vi "compile_table.vi"(6 "income_array":dbl[][](array[numeric]), 7 "row_number":i32, 8 "error_in":errorcluster, 9 "value":dbl, 10 "boc-data":sgl[](array[numeric]), 11 "measured":dbl[](array[numeric])) -> (0 "error_out":errorcluster, 2 "table":string[][](array[string]), 3 "output_data":dbl[][](array[numeric]))   [LabVIEW 2017]
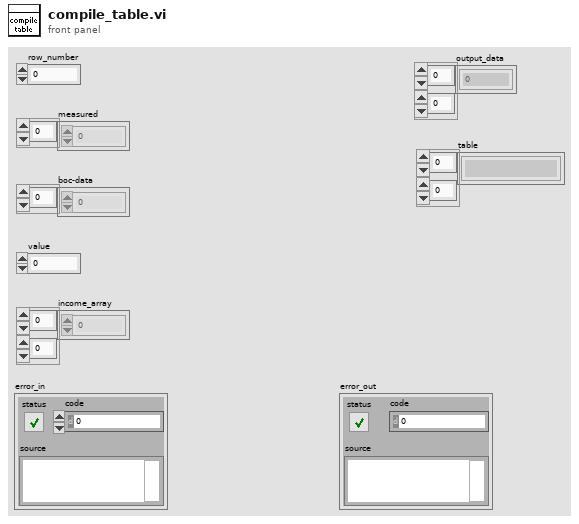
[diagram p1: front panel]
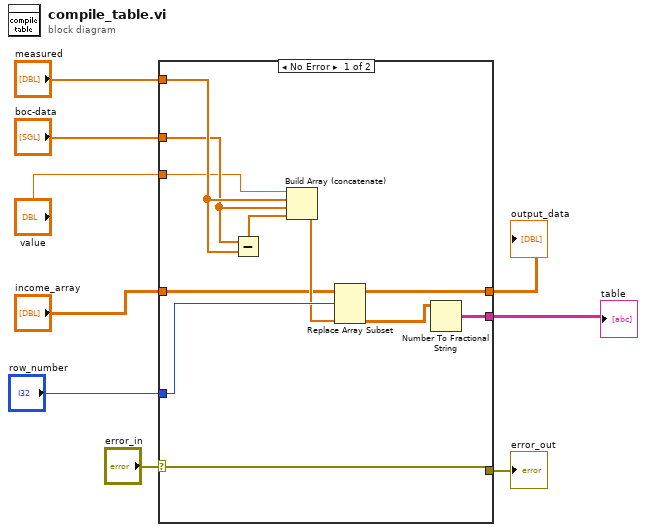
[diagram p0: block diagram]
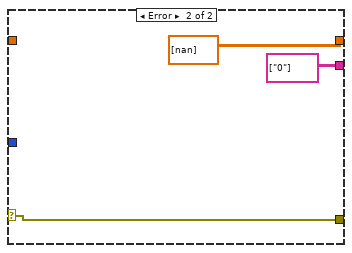
[diagram p2: hidden frame]
diagram:
  n1 = case shown="No Error" "error_in" {
    selector: "error_in" -> [w12 w22]
    tunnel: "measured" -> [w19 _]
    tunnel: "boc-data" -> [w18 _]
    tunnel: "row_number" -> [w16 _]
    tunnel: [w10 dbl[][] [[nan]] ("income_array")] -> w6
    tunnel: [w11 string[][] [["0"]]] -> w5
    tunnel: "income_array" -> [w14 _]
    tunnel: "value" -> [w13 _]
    tunnel: [w12 w22] -> w2
    frame No Error {
      n2 = Subtract(x=w18, y=w19) -> (x-y=w17:dbl[])
      n3 = Build Array (concatenate)(w13, w19, w18, w17) -> (w15:dbl[])
      n4 = Replace Array Subset(array=w14, new element=w15, index (row)=w16) -> (w10:dbl[][])  [unwired: 1 in]
      n5 = Number To Fractional String(number=w10) -> (F-format string=w11:string[][])  [unwired: 3 in]
    }
    frame Error {
    }
  }
  "output_data" <- w6
  "table" <- w5
  "error_out" <- w2
